vi "Disdrometer_WriteConfigFile.vi"(8 "ErrorIn":errorcluster, 11 "User":T1={"Port"="Port2", "SNR Threshold"=0.0, "FileFolder"=path "C:/ConnexData"}) -> (0 "ErrorOut":errorcluster)   [LabVIEW 2018]
doc: "Write the configuration (INI) file specified in ClusterIn.Paths.CfgFile. Add elements to this VI for each cluster element that you wish to save.\n\nCopyright © 2019 Epimedia, Inc. All Rights Reserved.\n\nThe Epimedia Application Library is Copyright © 2009-2017 Epimedia, Inc. \nAll Rights Reserved. Used under license."
uses:
  Disdrometer_UserDefined_clust.ctl
  <vilib>/Utility/sysdir.llb/System Directory Type.ctl
  <vilib>/Utility/xml.llb/Write to XML File(string).vi
panel:
  # "Copyright © 2019 Epimedia, Inc. All Rights Reserved.\n\nThe Epimedia Application Library is Copyright © 2009-2017 Epimedia, Inc. \nAll Rights Reserved. Used under license."
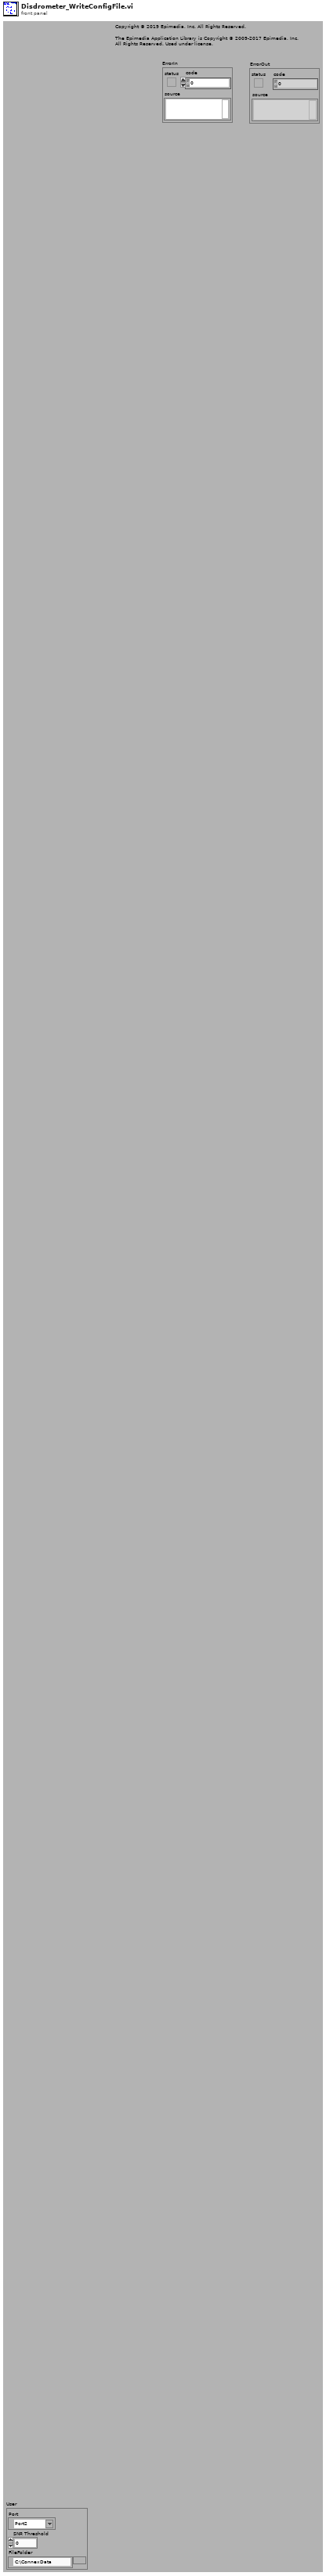
[diagram p1: front panel]
types:
  T1 = typedef "Disdrometer_UserDefined_clust.ctl" = cluster{"Port":refnum<visa-resource-name>, "SNR Threshold":dbl, "FileFolder":path}
  T2 = typedef "System Directory Type.ctl" = i32
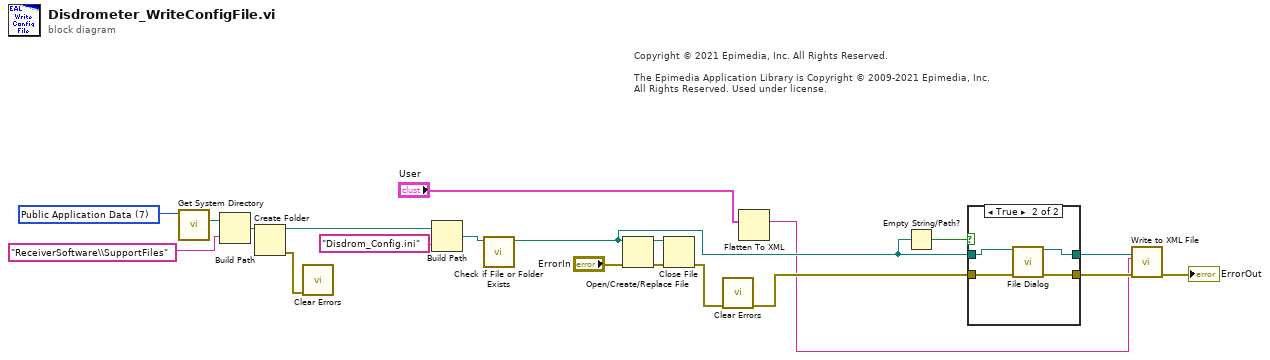
[diagram p0: block diagram]
diagram:
  w14 = T2 7 items=["User Home"=0, "User Desktop"=1, "User Documents"=2, "User Application Data"=3, "User Preferences"=4, "User Temporary"=5, "Public Documents"=6, "Public Application Data"=7, "Public Preferences"=8, "Public Cache"=13, "System Core Libraries"=9, "System Installed Libraries"=10, "Application Files"=11, "Boot Volume Root"=12] ("system directory type")
  # "Copyright © 2021 Epimedia, Inc. All Rights Reserved.\n\nThe Epimedia Application Library is Copyright © 2009-2021 Epimedia, Inc. \nAll Rights Reserved. Used under license."
  n1 = call <vilib>:"Get System Directory.vi"("system directory type"=w14) -> ("system directory"=w16:path)  [unwired: 10 in]
  n2 = Build Path(base path=w16, name or relative path="ReceiverSoftware\\SupportFiles") -> (appended path=w17:path)
  n3 = Create Folder(path (use dialog)=w17) -> (created path=w13:path, error out=w1:errorcluster)  [unwired: 2 in, 1 out]
  n4 = call <vilib>:"Clear Errors.vi"("error in (no error)"=w1) -> ()  [unwired: 5 in, 2 out]
  n5 = Build Path(base path=w13, name or relative path="Disdrom_Config.ini") -> (appended path=w12:path)
  n6 = call <vilib>:"Check if File or Folder Exists.vi"("path"=w12) -> ("dup path"=w11:path)  [unwired: 1 in, 9 out]
  n7 = Open/Create/Replace File(file path (use dialog)=w11, error in="ErrorIn") -> (refnum out=w10:refnum<file>, error out=w9:errorcluster)  [unwired: 4 in, 1 out]
  n8 = Close File(refnum=w10, error in=w9) -> (error out=w8:errorcluster)  [unwired: 1 out]
  n9 = call <vilib>:"Clear Errors.vi"("error in (no error)"=w8) -> ("error out"=w6:errorcluster)  [unwired: 5 in, 1 out]
  n10 = Flatten To XML(anything="User") -> (xml string=w3:string)
  n11 = Empty String/Path?(string/path=w11) -> (empty?=w7:bool)
  n12 = case shown="True" w7 {
    tunnel: w11 -> [w21 w26]
    tunnel: w6 -> [w22 w25]
    tunnel: [w22 w24] -> w5
    tunnel: [w21 w23] -> w4
    frame False {
    }
    frame True {
      n13 = call "File Dialog"("start path"=w26, "error in"=w25) -> ("selected path"=w23:path, "error out"=w24:errorcluster)  [unwired: 10 in, 2 out]
    }
  }
  n14 = call-poly <vilib>:"Write to XML File.vi"("error in (no error)"=w5, "XML Input"=w3, "XML File Path"=w4) -> ("error out"=→"ErrorOut":errorcluster)  [unwired: 6 in, 2 out]
